vi "_concat_mode_control.vi"(10 "write buffer":string, 11 "[x]":T1) -> (2 "write buffer out":string)   [LabVIEW 2023, in "Chemyx_Syringe_Pump_driver.lvlib"]
uses:
  Chemyx_Syringe_Pump_driver.lvlib
  Control/Control Mode.ctl
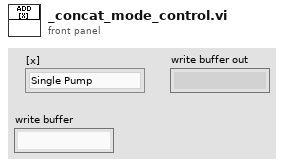
[diagram p1: front panel]
types:
  T1 = typedef "Chemyx_Syringe_Pump_driver.lvlib/Control Mode.ctl" = enum16{"Single Pump", "Pump Channel 1", "Pump Channel 2", "Cycle Mode"}
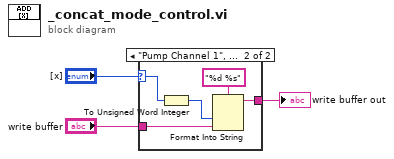
[diagram p0: block diagram]
diagram:
  n1 = case shown="\"Pump Channel 1\", Default" "[x]" {
    selector: "[x]" -> [_ w9]
    tunnel: [w4 w5] -> w1
    tunnel: "write buffer" -> [w4 w8]
    frame "Single Pump" {
    }
    frame "Pump Channel 1", Default {
      n2 = To Unsigned Word Integer(number=w9) -> (unsigned 16bit integer=w7:u16)
      n3 = Format Into String(format string="%d %s", w7, w8) -> (resulting string=w5:string)  [unwired: 2 in, 1 out]
    }
  }
  "write buffer out" <- w1
